vi "Close Artifactory.vi"(8 "error in (no error)":errorcluster, 11 "Artifactory in":refnum<class "Artifactory.lvclass">) -> (0 "error out":errorcluster, 3 "Artifactory out":refnum<class "Artifactory.lvclass">)   [LabVIEW 2021, in "Artifactory.lvclass"]
uses:
  Artifactory.lvclass
  Artifactory.lvclass/Artifactory.ctl
  <vilib>/addons/_JKI.lib/REST Client/classes/REST Client/REST Client.lvclass
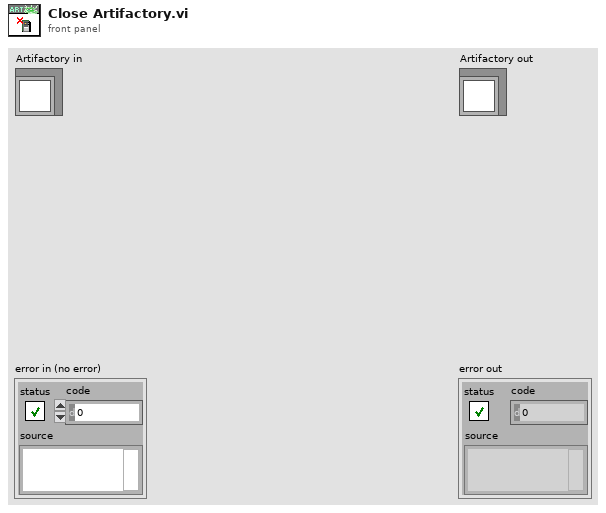
[diagram p1: front panel]
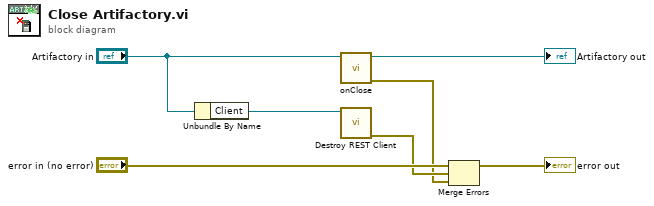
[diagram p0: block diagram]
diagram:
  n1 = Unbundle By Name("Artifactory in") -> ("Client"=w5:refnum<class "REST Client.lvclass">)
  n2 = call-dynamic "onClose.vi"("Artifactory in"="Artifactory in") -> ("error out"=w1:errorcluster, "Artifactory out"=→"Artifactory out":refnum<class "Artifactory.lvclass">)  [unwired: 9 in]
  n3 = call-dynamic "Destroy REST Client.vi"("REST Client in"=w5) -> ("error out"=w4:errorcluster)  [unwired: 10 in]
  n4 = Merge Errors("error in (no error)", w4, w1) -> (→"error out":errorcluster)
